vi "App enquece opposite.vi"(8 "error in (no error)":errorcluster, 9 "command data":variant, 10 "command":string="INIT.Read HW config", 11 "Queue in":refnum<queue>) -> (0 "error out":errorcluster, 3 "queue out":refnum<queue>)   [LabVIEW 2018]
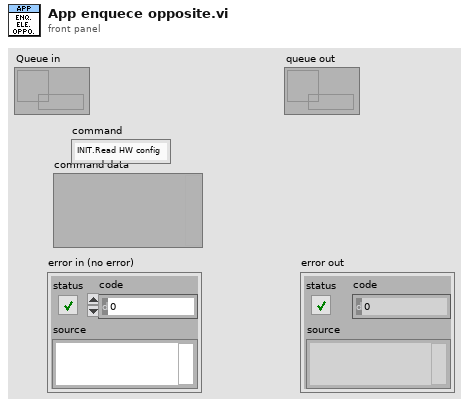
[diagram p1: front panel]
types:
  T1 = cluster{"command":string, "command data":variant}
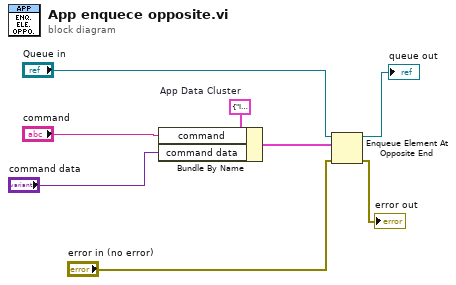
[diagram p0: block diagram]
diagram:
  w4 = T1 {"command"="INIT.Read HW config", "command data"=variant}  # App Data Cluster
  n1 = Bundle By Name(cluster=w4, "command"="command", "command data"="command data") -> (w8:T1)
  n2 = Enqueue Element At Opposite End(queue="Queue in", element=w8, error in (no error)="error in (no error)") -> (queue out=→"queue out":refnum<queue>, error out=→"error out":errorcluster)  [unwired: 1 in, 1 out]
